vi "DSF.Engine.Framework.Tx.vi"(8 "error in (no error)":errorcluster, 11 "Framework in":refnum<class "DSF.Engine.Framework.lvclass">) -> (0 "error out":errorcluster, 3 "Framework out":refnum<class "DSF.Engine.Framework.lvclass">)   [LabVIEW 2017, in "DSF.Engine.lvlib" / "DSF.Engine.Framework.lvclass"]
uses:
  DSF.Engine.Framework.lvclass
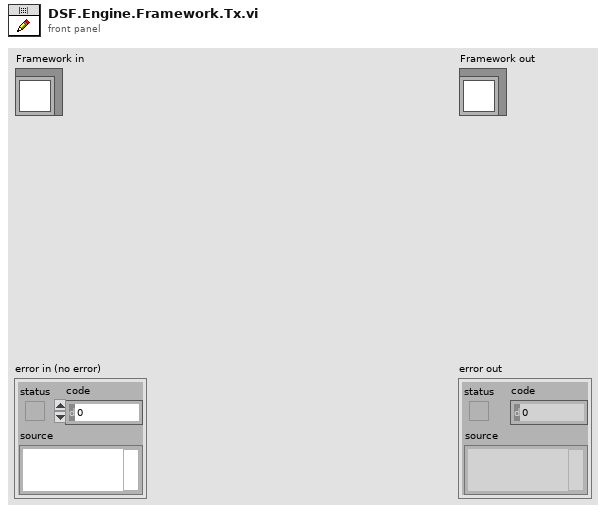
[diagram p1: front panel]
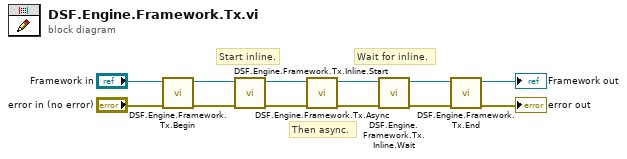
[diagram p0: block diagram]
diagram:
  # "Wait for inline."
  # "Start inline."
  # "Then async."
  n1 = call "DSF.Engine.Framework.Tx.Begin.vi"("error in (no error)"="error in (no error)", "Framework in"="Framework in") -> ("error out"=w5:errorcluster, "Framework out"=w6:refnum<class "DSF.Engine.Framework.lvclass">)  [unwired: 8 in]
  n2 = call "DSF.Engine.Framework.Tx.Inline.Start.vi"("error in (no error)"=w5, "Framework in"=w6) -> ("error out"=w10:errorcluster, "Framework out"=w9:refnum<class "DSF.Engine.Framework.lvclass">)  [unwired: 8 in]
  n3 = call "DSF.Engine.Framework.Tx.Async.vi"("error in (no error)"=w10, "Framework in"=w9) -> ("error out"=w12:errorcluster, "Framework out"=w11:refnum<class "DSF.Engine.Framework.lvclass">)  [unwired: 8 in]
  n4 = call "DSF.Engine.Framework.Tx.Inline.Wait.vi"("error in (no error)"=w12, "Framework in"=w11) -> ("error out"=w3:errorcluster, "Framework out"=w4:refnum<class "DSF.Engine.Framework.lvclass">)  [unwired: 8 in]
  n5 = call "DSF.Engine.Framework.Tx.End.vi"("error in (no error)"=w3, "Framework in"=w4) -> ("error out"=→"error out":errorcluster, "Framework out"=→"Framework out":refnum<class "DSF.Engine.Framework.lvclass">)  [unwired: 8 in]
